vi "Insert Element at Start.vi"(0 "Variant (Cluster) in":variant, 5 "Name":string, 7 "element":variant, 11 "error in (no error)":errorcluster) -> (4 "Variant (Cluster) out":variant, 15 "error out":errorcluster)   [LabVIEW 2017, in "Advanced Variant Tools.lvlib"]
uses:
  Advanced Variant Tools.lvlib
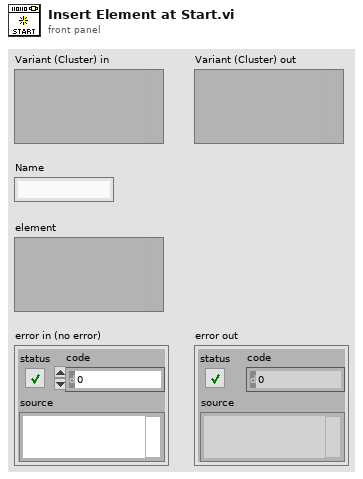
[diagram p1: front panel]
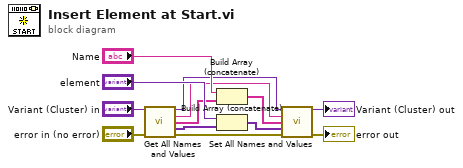
[diagram p0: block diagram]
diagram:
  n1 = call "Get All Names and Values.vi"("Variant (Cluster) In"="Variant (Cluster) in", "error in"="error in (no error)") -> ("Variant (Cluster) Out"=w1:variant, "Name"=w2:string, "Element Names"=w5:string[], "Values"=w12:variant[], "error out"=w11:errorcluster)  [unwired: 9 in]
  n2 = Build Array (concatenate)("Name", w5) -> (w3:string[])
  n3 = Build Array (concatenate)("element", w12) -> (w8:variant[])
  n4 = call "Set All Names and Values.vi"("Variant (Cluster) In"=w1, "Name"=w2, "Element Names"=w3, "values"=w8, "error in"=w11) -> ("Variant (Cluster) Out"=→"Variant (Cluster) out":variant, "error out"=→"error out":errorcluster)  [unwired: 9 in]
